vi "Pathfiles.vi"() -> ()   [LabVIEW 2017]
panel:
  out "Log File Path":path
  out "Application Directory":path
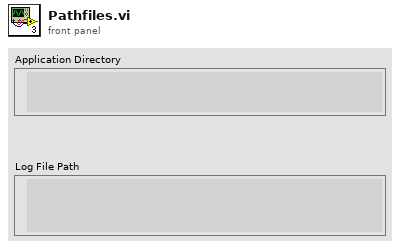
[diagram p1: front panel]
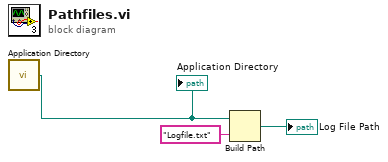
[diagram p0: block diagram]
diagram:
  n1 = call <vilib>:"Application Directory.vi"() -> ("Application Directory"=w3:path)
  "Application Directory" <- w3
  n2 = Build Path(base path=w3, name or relative path="Logfile.txt") -> (appended path=→"Log File Path":path)
